vi "Pozycjonuj_wolna.vi"(8 "error in (no error)":errorcluster, 10 "Pos Array":T1[](array[typedef]), 11 "Array":refnum<vi>[](array[refnum])) -> (0 "error out":errorcluster)   [LabVIEW 2014]
doc: "Pozycjonuje elementy znajdujace sie tylko w oknie Akwizycja Wolna"
uses:
  <vilib>/Utility/miscctls.llb/LVPositionTypeDef.ctl
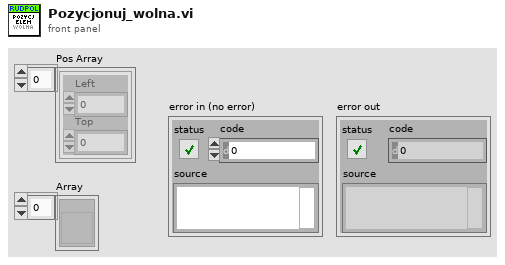
[diagram p1: front panel]
types:
  T1 = typedef "LVPositionTypeDef.ctl" = cluster{"Left":i32, "Top":i32}
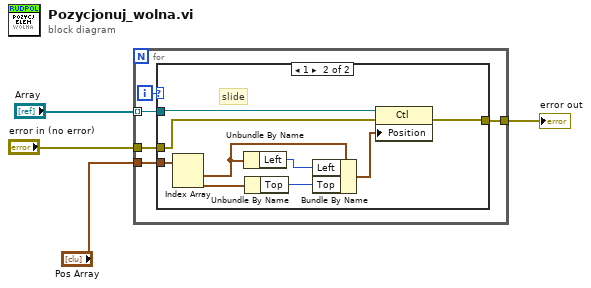
[diagram p0: block diagram]
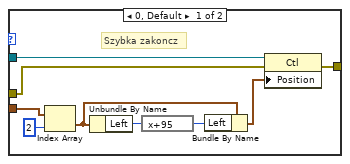
[diagram p2: hidden frame]
diagram:
  n1 = for {
    tunnel: "Array" -> [w7] mode=indexing
    tunnel: "Pos Array" -> [w8]
    tunnel: "error in (no error)" -> [w6]
    tunnel: [w5] -> w1
    i -> [w9]
    n2 = case shown="1" w9 {
      tunnel: w8 -> [w17 w26]
      tunnel: w7 -> [w18 w27]
      tunnel: w6 -> [w11 w19]
      tunnel: [w10 w20] -> w5
      frame 0, Default {
        # "Szybka zakoncz"
        n3 = Index Array(array=w17, index=2) -> (element=w15:T1)
        n4 = Unbundle By Name(w15) -> ("Left"=w13:i32)
        n5 = expression code="x+95"(w13) -> (w12:i32)
        n6 = Bundle By Name(cluster=w15, "Left"=w12) -> (w14:T1)
        n7 = property class="Ctl"(reference=w18, error in=w11, "Position"=w14) -> (error out=w10:errorcluster)  [unwired: 1 out]
      }
      frame 1 {
        # "slide"
        n8 = Index Array(array=w26) -> (element #1=w25:T1, element #2=w23:T1)  [unwired: 2 in]
        n9 = Unbundle By Name(w25) -> ("Left"=w22:i32)
        n10 = Unbundle By Name(w23) -> ("Top"=w21:i32)
        n11 = Bundle By Name(cluster=w25, "Left"=w22, "Top"=w21) -> (w24:T1)
        n12 = property class="Ctl"(reference=w27, error in=w19, "Position"=w24) -> (error out=w20:errorcluster)  [unwired: 1 out]
      }
    }
  }
  "error out" <- w1
